vi "Build.vi"(9 "XYZTheta":dbl[](array[numeric]), 10 "Pattern Coordinates":dbl[][](array[numeric]), 11 "CAD Dispense in":refnum<class "CAD Dispense.lvclass">) -> (3 "CAD Dispense out":refnum<class "CAD Dispense.lvclass">)   [LabVIEW 2020, in "CAD Dispense.lvclass"]
uses:
  CAD Dispense.lvclass
  <vilib>/Analysis/NI_AALPro.lvlib
  <vilib>/Analysis/coordinate.llb/2D Cartesian Coordinate Rotation (Scalar).vi
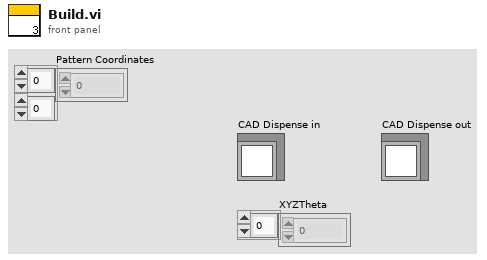
[diagram p1: front panel]
types:
  T1 = cluster{"Motion":dbl[][], "Center":dbl[], "CW/CCW":dbl, "Dispense Type":enum16{"N-gon", "Square", "Arc", "Dot", "Line", "Circle"}}[]
  T2 = cluster{"Motion":dbl[][], "Center":dbl[], "CW/CCW":dbl, "Dispense Type":enum16{"N-gon", "Square", "Arc", "Dot", "Line", "Circle"}}
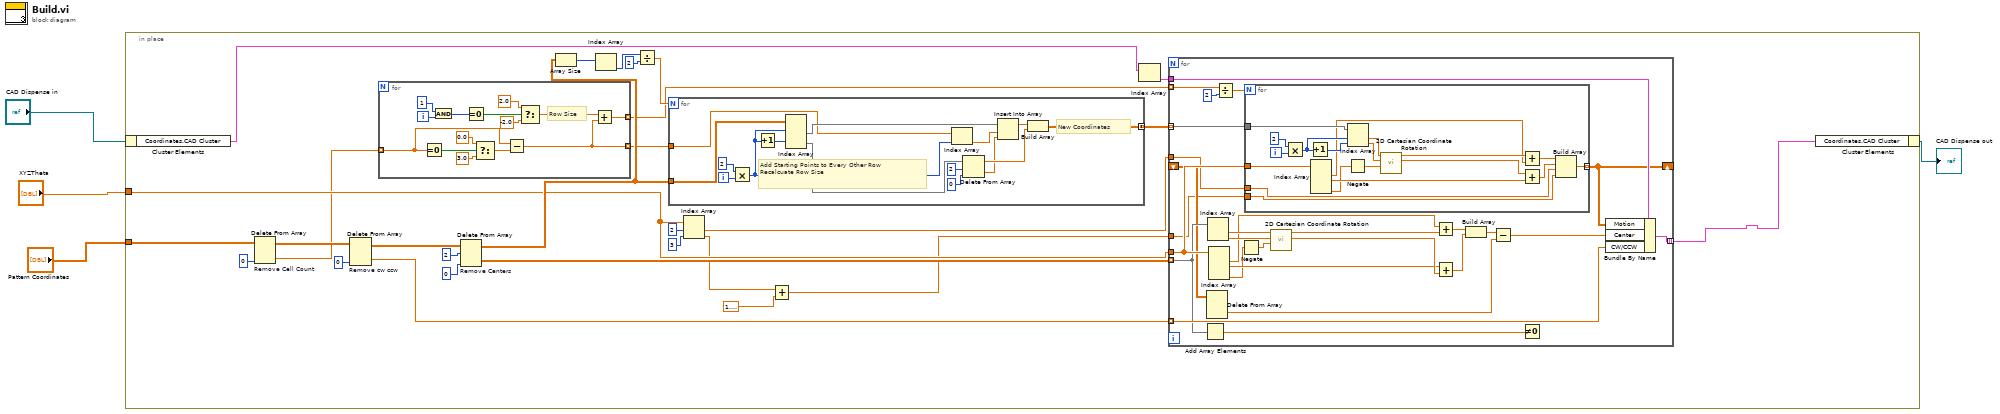
[diagram p0: block diagram]
diagram:
  n1 = in-place {
    in-place-border: "XYZTheta" -> [w13]
    in-place-border: "Pattern Coordinates" -> [w19]
    n2 = in-place-cluster #1("CAD Dispense in") -> ("Coordinates.CAD Cluster"=w21:T1)
    n3 = Delete From Array "Remove Cell Count"(array=w19, index (col)=0 ("disabled index (col)")) -> (deleted portion=w6:dbl[], array with subset deleted=w26:dbl[][])  [unwired: 2 in]
    n4 = Delete From Array "Remove cw ccw"(array=w26, index (col)=0 ("disabled index (col)")) -> (deleted portion=w31:dbl[], array with subset deleted=w27:dbl[][])  [unwired: 2 in]
    n5 = for {
      tunnel: w6 -> [w42] mode=indexing
      tunnel: [w34] -> w15 mode=indexing
      tunnel: [w33] -> w14 mode=indexing
      i -> [w35]
      # "Row Size"
      n6 = Equal To 0?(x=w42) -> (x = 0?=w43:bool)
      n7 = And(x=1, y=w35) -> (x .and. y?=w38:i32)
      n8 = Equal To 0?(x=w38) -> (x = 0?=w36:bool)
      n9 = Select(t=0.0, s=w43, f=3.0) -> (s? t:f=w46:dbl)
      n10 = Subtract(x=w42, y=w46) -> (x-y=w33:dbl)
      n11 = Select(t=2.0, s=w36, f=-2.0) -> (s? t:f=w39:dbl)
      n12 = Add(x=w39, y=w33) -> (x+y=w34:dbl)
    }
    n13 = Delete From Array "Remove Centers"(array=w27, length=2, index (col)=0 ("disabled index (col)")) -> (deleted portion=w32:dbl[][], array with subset deleted=w28:dbl[][])  [unwired: 1 in]
    n14 = Array Size(array=w28) -> (size(s)=w29:i32[])
    n15 = Index Array(array=w29) -> (element=w18:i32)  [unwired: 1 in]
    n16 = Divide(x=w18, y=2) -> (x/y=w16:dbl)
    n17 = for {
      N: w16 -> [_]
      tunnel: w28 -> [w107]
      tunnel: [w99] -> w30 mode=concatenating
      tunnel: w14 -> [w94]
      i -> [w100]
      # "New Coordinates"
      # "Add Starting Points to Every Other Row\nRecalcuate Row Size"
      n18 = Multiply(x=2, y=w100) -> (x*y=w93:i32)
      n19 = Increment(x=w93) -> (x+1=w95:i32)
      n20 = Index Array(array=w107, index (row) #1=w93, index (row) #2=w95) -> (element #1=w103:dbl[], element #2=w105:dbl[])  [unwired: 2 in]
      n21 = Index Array(array=w94, index=w93) -> (element=w96:dbl)
      n22 = Delete From Array(array=w105, length=2, index=0) -> (deleted portion=w97:dbl[], array with subset deleted=w101:dbl[])
      n23 = Insert Into Array(array=w103, index=w96, new element=w97) -> (w102:dbl[])
      n24 = Build Array(w102, w101) -> (w99:dbl[][])
    }
    n25 = Index Array(array=w13, index #1=2 ("index"), index #2=3 ("index")) -> (element #1=w8:dbl, element #2=w9:dbl)
    n26 = Add(x=w9, y=1.5707963267948966) -> (x+y=w7:dbl)
    n27 = Index Array(array=w21) -> (element=w20:T2)  [unwired: 1 in]
    n28 = for {
      tunnel: w15 -> [w71] mode=indexing
      tunnel: w30 -> [w67] mode=indexing
      tunnel: w31 -> [w69] mode=indexing
      tunnel: w32 -> [w66] mode=indexing
      tunnel: w13 -> [w72]
      tunnel: w20 -> [w70]
      tunnel: [w68] -> w5 mode=indexing
      shift-right: [w49] -> _
      shift-left: _ -> [w55]
      tunnel: w7 -> [w47]
      tunnel: w8 -> [w48]
      n29 = Add Array Elements(numeric array=w66) -> (sum=w52:dbl)
      n30 = Delete From Array(array=w55) -> (deleted portion=w54:dbl[])  [unwired: 3 in, 1 out]
      n31 = Index Array(array=w66) -> (element #1=w65:dbl, element #2=w64:dbl)  [unwired: 2 in]
      n32 = Index Array(array=w72) -> (element #1=w62:dbl, element #2=w57:dbl, element #4=w51:dbl)  [unwired: 4 in, 1 out]
      n33 = Divide(x=w71, y=2) -> (x/y=w63:dbl)
      n34 = Negate(x=w51) -> (-x=w50:dbl)
      n35 = for {
        N: w63 -> [_]
        tunnel: w67 -> [w92]
        tunnel: [w78] -> w49 mode=indexing
        tunnel: w72 -> [w88]
        tunnel: w48 -> [w75]
        tunnel: w47 -> [w74]
        i -> [w79]
        n36 = Multiply(x=2, y=w79) -> (x*y=w90:i32)
        n37 = Increment(x=w90) -> (x+1=w89:i32)
        n38 = Index Array(array=w88) -> (element #1=w81:dbl, element #2=w80:dbl, element #4=w77:dbl)  [unwired: 4 in, 1 out]
        n39 = Negate(x=w77) -> (-x=w76:dbl)
        n40 = Index Array(array=w92, index #1=w90, index #2=w89) -> (element #1=w84:dbl, element #2=w83:dbl)
        n41 = call-poly <vilib>:"2D Cartesian Coordinate Rotation.vi"("theta"=w76, "y"=w83, "x"=w84) -> ("y out"=w87:dbl, "x out"=w82:dbl)  [unwired: 6 in, 1 out]
        n42 = Add(x=w82, y=w81) -> (x+y=w86:dbl)
        n43 = Add(x=w87, y=w80) -> (x+y=w85:dbl)
        n44 = Build Array(w86, w85, w75, w74) -> (w78:dbl[])
      }
      n45 = call-poly <vilib>:"2D Cartesian Coordinate Rotation.vi"("theta"=w50, "y"=w64, "x"=w65) -> ("y out"=w59:dbl, "x out"=w61:dbl)  [unwired: 6 in, 1 out]
      n46 = Add(x=w62, y=w61) -> (x+y=w60:dbl)
      n47 = Add(x=w57, y=w59) -> (x+y=w58:dbl)
      n48 = Build Array(w60, w58) -> (w56:dbl[])
      n49 = Subtract(x=w56, y=w54) -> (x-y=w53:dbl[])
      n50 = Not Equal To 0?(x=w52) -> ()  [unwired: 1 out]
      n51 = Bundle By Name(cluster=w70, "Motion"=w49, "Center"=w53, "CW/CCW"=w69) -> (w68:T2)
    }
    n52 = in-place-cluster #1("Coordinates.CAD Cluster"=w5) -> (→"CAD Dispense out":refnum<class "CAD Dispense.lvclass">)
  }
